vi "SMTP Email SJIS To JIS.vi"(0 "text in":string) -> (4 "text out":string)   [LabVIEW 2011, in "NewNI_SMTPEmail.lvlib"]
uses:
  NewNI_SMTPEmail.lvlib
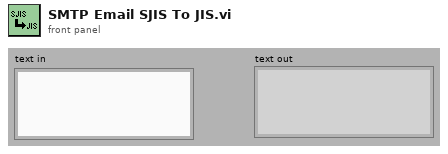
[diagram p1: front panel]
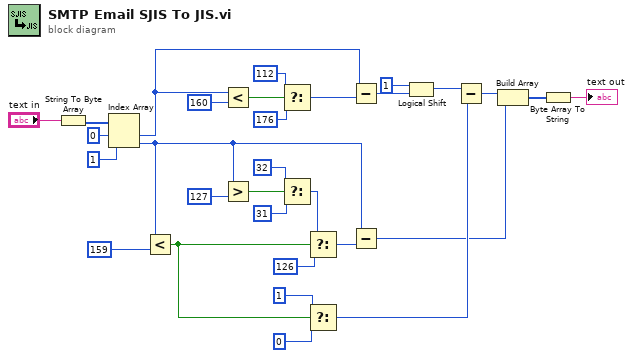
[diagram p0: block diagram]
diagram:
  n1 = String To Byte Array(string="text in") -> (unsigned byte array=w29:u8[])
  n2 = Index Array(array=w29, index #1=0 ("index"), index #2=1 ("index")) -> (element #1=w14:u8, element #2=w5:u8)
  n3 = Less?(x=w5, y=u8 159) -> (x < y?=w10:bool)
  n4 = Less?(x=w14, y=u8 160) -> (x < y?=w24:bool)
  n5 = Greater?(x=w5, y=u8 127) -> (0:w17:bool)
  n6 = Select(t=u8 112 ("y"), s=w24, f=u8 176 ("y")) -> (s? t:f=w15:u8)
  n7 = Select(t=u8 32 ("y"), s=w17, f=u8 31 ("y")) -> (s? t:f=w16:u8)
  n8 = Select(t=w16, s=w10, f=u8 126 ("y")) -> (s? t:f=w6:u8)
  n9 = Select(t=u8 1 ("y"), s=w10, f=u8 0 ("y")) -> (s? t:f=w7:u8)
  n10 = Subtract(x=w14, y=w15) -> (x-y=w13:u8)
  n11 = Subtract(x=w5, y=w6) -> (x-y=w3:u8)
  n12 = Logical Shift(y=u8 1, x=w13) -> (x << y=w11:u8)
  n13 = Subtract(x=w11, y=w7) -> (x-y=w4:u8)
  n14 = Build Array(w4, w3) -> (w2:u8[])
  n15 = Byte Array To String(unsigned byte array=w2) -> (string=→"text out":string)
